vi "SensorRead.vi"() -> ()   [LabVIEW 2012]
uses:
  Robot Global Data.vi
panel:
  in  "ResetLauncherGyro":bool
  in  "ResetRobotGyro":bool
  out "LauncherGyroAngle":dbl
  out "RobotGyroAngle":dbl
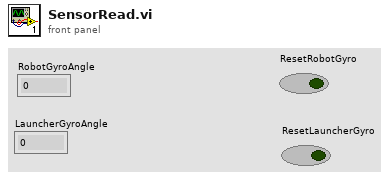
[diagram p1: front panel]
types:
  T1 = typedef "WPI_GyroDevRef.ctl" = cluster{"DevStatus":errorcluster, "Analog Module":T2, "Analog Channel":T3, "Offset":dbl, "Gain (VoltsPerDegree/Second)":dbl}
  T2 = typedef "FPGA_TypedefAnalogModule.ctl" = enum16{"Analog Module 1", "Analog Module 2"}
  T3 = typedef "FPGA_AIChannel.ctl" = enum8{"AI 1", "AI 2", "AI 3", "AI 4", "AI 5", "AI 6", "AI 7", "AI 8", "Invalid"}
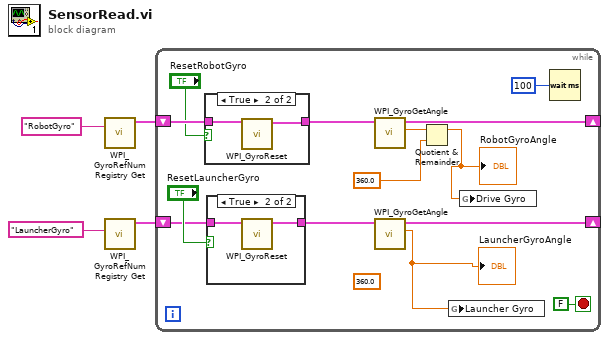
[diagram p0: block diagram]
diagram:
  n1 = call <vilib>:"WPI_GyroRefNum Registry Get.vi"("refnum name"="RobotGyro") -> ("GyroDevRef"=w3:T1)  [unwired: 9 in, 1 out]
  n2 = call <vilib>:"WPI_GyroRefNum Registry Get.vi"("refnum name"="LauncherGyro") -> ("GyroDevRef"=w1:T1)  [unwired: 9 in, 1 out]
  n3 = while {
    shift-right: [w18] -> _
    shift-left: w3 -> [w11]
    shift-right: [w13] -> _
    shift-left: w1 -> [w8]
    stop <- FALSE stop-if-true
    (unwired) 360.0
    n4 = case shown="True" "ResetRobotGyro" {
      tunnel: [w22 w23] -> w12
      tunnel: w11 -> [w22 w24]
      frame False {
      }
      frame True {
        n5 = call <vilib>:"WPI_GyroReset.vi"("GyroDevRef"=w24) -> ("GyroDevRef"=w23:T1)  [unwired: 9 in, 1 out]
      }
    }
    n6 = case shown="True" "ResetLauncherGyro" {
      tunnel: w8 -> [w19 w21]
      tunnel: [w19 w20] -> w7
      frame False {
      }
      frame True {
        n7 = call <vilib>:"WPI_GyroReset.vi"("GyroDevRef"=w21) -> ("GyroDevRef"=w20:T1)  [unwired: 9 in, 1 out]
      }
    }
    n8 = call <vilib>:"WPI_GyroGetAngle.vi"("GyroDevRef"=w12) -> ("Angle"=w14:dbl, "GyroDevRef"=w18:T1)  [unwired: 7 in, 2 out]
    n9 = call <vilib>:"WPI_GyroGetAngle.vi"("GyroDevRef"=w7) -> ("Angle"=w5:dbl, "GyroDevRef"=w13:T1)  [unwired: 7 in, 2 out]
    "LauncherGyroAngle" <- w5
    n10 = Quotient & Remainder(x=w14, y=360.0) -> (x-y*floor(x/y)=w6:dbl)  [unwired: 1 out]
    "RobotGyroAngle" <- w6
    n11 = global write "Robot Global Data.vi" "Launcher Gyro"(w5) -> ()
    n12 = global write "Robot Global Data.vi" "Drive Gyro"(w6) -> ()
    n13 = Wait (ms)(milliseconds to wait=u32 100) -> ()  [unwired: 1 out]
  }
